vi "niScope Set DDC Filter Coefficients.vi"(0 "instrument handle":refnum<k15>, 5 "channels":string="0", 7 "coefficient type":enum16{"Programmable FIR", "Discriminator FIR"}(ring), 9 "coefficients":i32[](array[numeric])=[-2147483648, 0, 0, 0, 0, 0, 0, 0, 0, 0, 0, 0, 0, 0, 0, 0, 0, 0, 0, 0, 0, 0, 0, 0, 0, 0, 0, 0, 0, 0, 0, 0, 0, 0, 0, 0, 0, 0, 0, 0, 0, 0, 0, 0, 0, 0, 0, 0, 0, 0, 0, 0, 0, 0, 0, 0, 0, 0, 0, 0, 0, 0, 0, 0, 0, 0, 0, 0, 0, 0, 0, 0, 0, 0, 0, 0, 0, 0, 0, 0, 0, 0, 0, 0, 0, 0, 0, 0, 0, 0, 0, 0, 0, 0, 0, 0, 0, 0, 0, 0, 0, 0, 0, 0, 0, 0, 0, 0, 0, 0, 0, 0, 0, 0, 0, 0, 0, 0, 0, 0, 0, 0, 0, 0, 0, 0, 0, 0] format="%.0x", 11 "error in":errorcluster) -> (4 "instrument handle out":refnum<k15>, 15 "error out":errorcluster)   [LabVIEW 2011]
doc: "Downloads programmable FIR and discriminator FIR filter coefficients to the digital downconverter (DDC) in the NI 5620/5621."
uses:
  niScope_32.dll
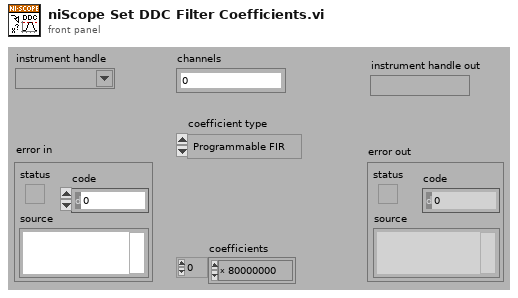
[diagram p1: front panel]
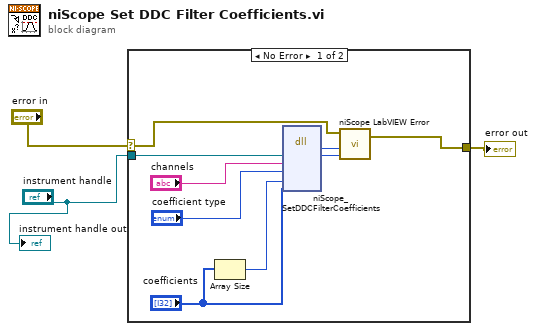
[diagram p0: block diagram]
diagram:
  n1 = case shown="No Error" "error in" {
    selector: "error in" -> [w4 w13]
    tunnel: [w9 w13] -> w3
    tunnel: "instrument handle" -> [w12 _]
    frame No Error {
      n2 = Array Size(array="coefficients") -> (size(s)=w5:i32)
      n3 = dll-call lib="niScope_*.*" fn="niScope_SetDDCFilterCoefficients"("instrument handle"=w12, "channel"="channels", "coefficientType"="coefficient type", "numCoefficients"=w5, "coefficients"="coefficients") -> ("status"=w11:i32, "instrument handle"=w10:u32)  [unwired: 7 in, 2 out]
      n4 = call <instrlib>:"niScope LabVIEW Error.vi"("instrument handle"=w10, "niScope error code (0)"=w11, "error in (no error)"=w4) -> ("error out"=w9:errorcluster)  [unwired: 2 in]
    }
    frame Error {
    }
  }
  "error out" <- w3
  "instrument handle out" <- "instrument handle"
